vi "FMV - click on control.vi"(8 "error in (no error)":errorcluster, 10 "Reference to Button":refnum<vi>, 11 "VI Reference":refnum<vi>) -> (0 "error out":errorcluster)   [LabVIEW 2020, in "ui-testing.lvlib"]
uses:
  ui-testing.lvlib
  User32.dll
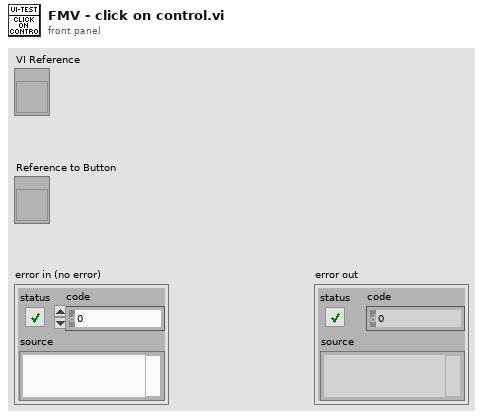
[diagram p1: front panel]
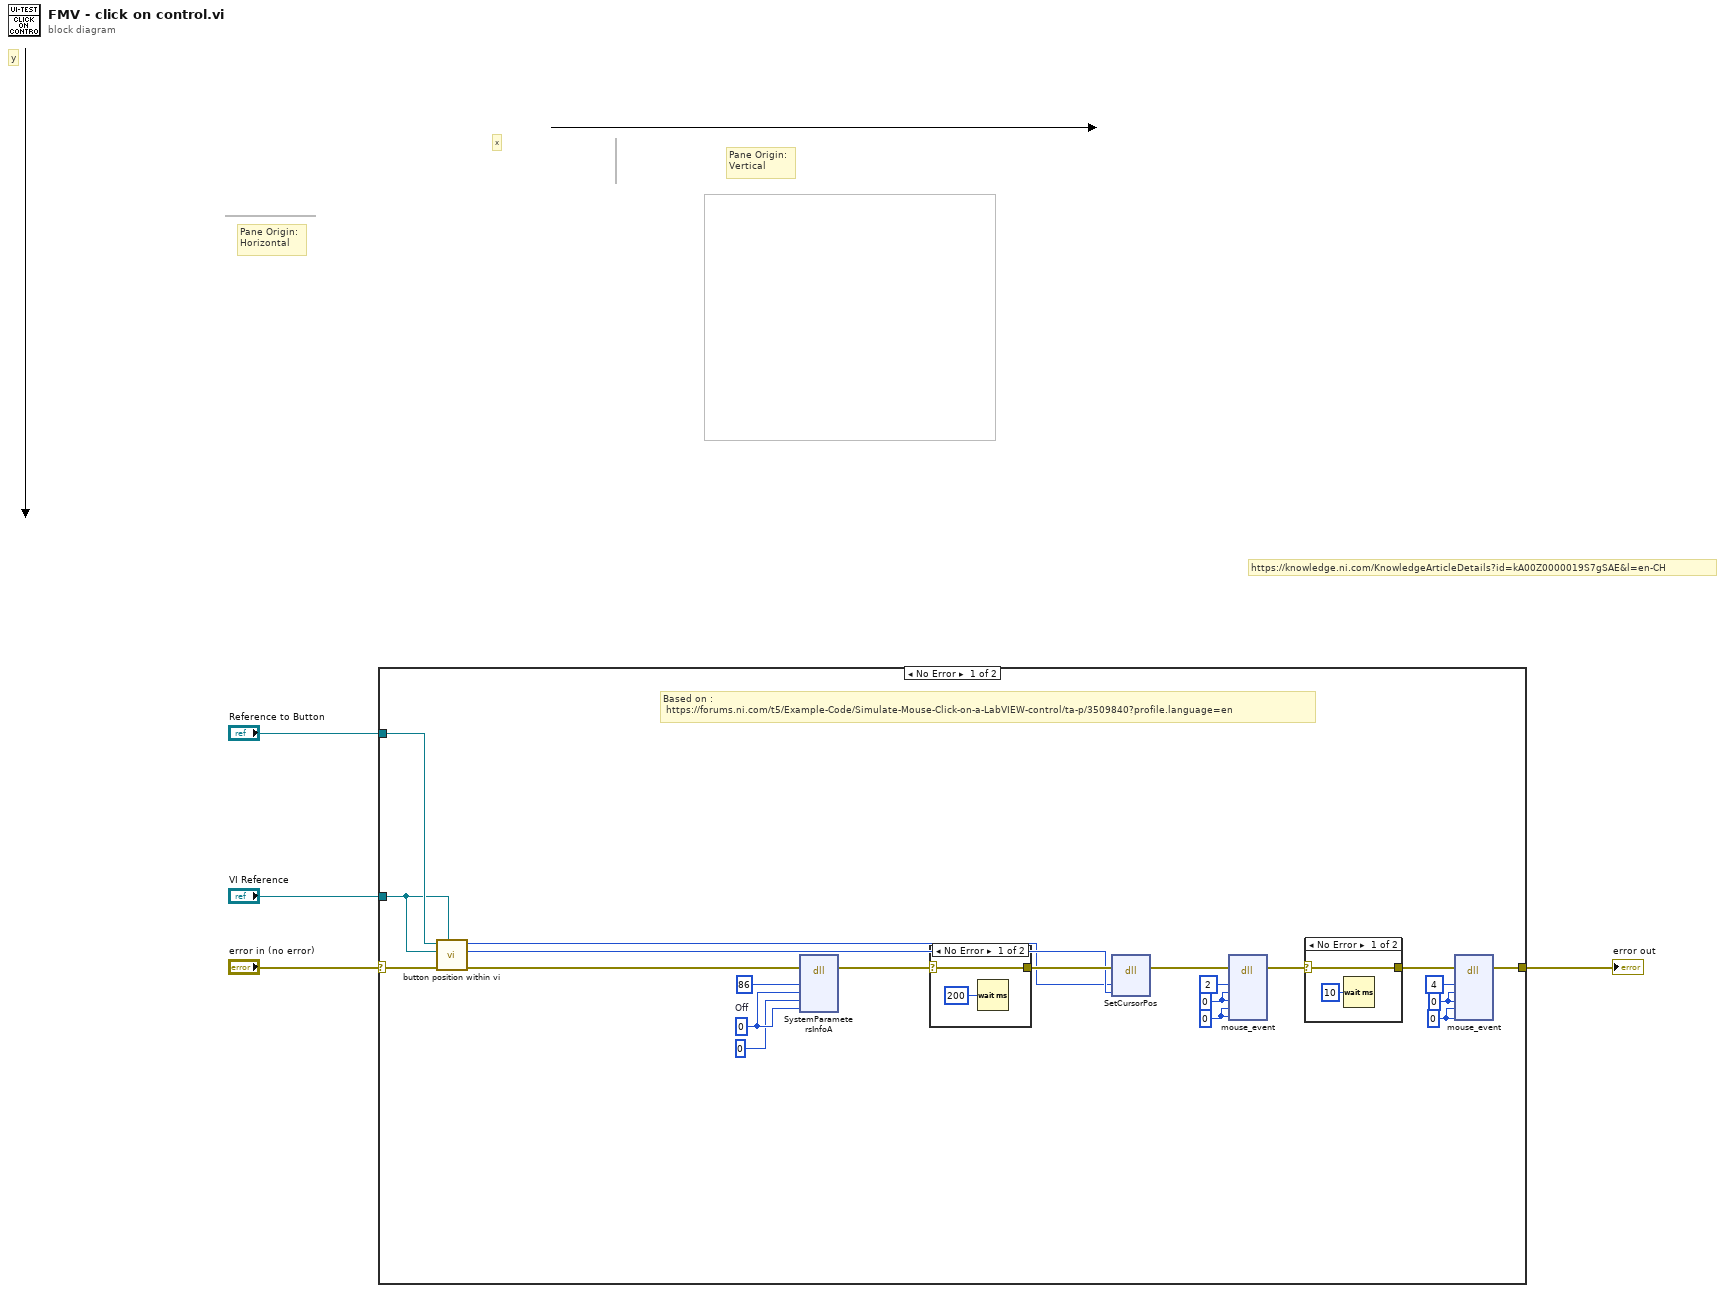
[diagram p0: block diagram]
diagram:
  # "https://knowledge.ni.com/KnowledgeArticleDetails?id=kA00Z0000019S7gSAE&l=en-CH"
  # "Pane Origin:\nVertical"
  # "Pane Origin:\nHorizontal"
  # "y"
  # "x"
  n1 = case shown="No Error" "error in (no error)" {
    selector: "error in (no error)" -> [w8 w32]
    tunnel: [w11 w32] -> w4
    tunnel: "Reference to Button" -> [w6 _]
    tunnel: "VI Reference" -> [w5 _]
    frame No Error {
      w23 = 0 ("dwExtraInfo")
      w24 = u32 0 ("dwExtraInfo")
      w22 = 0 ("dwExtraInfo")
      w21 = u32 0 ("dwExtraInfo")
      w19 = u32 0  # Off
      # "Based on :\n https://forums.ni.com/t5/Example-Code/Simulate-Mouse-Click-on-a-LabVIEW-control/ta-p/3509840?profile.language=en"
      n2 = call "button position within vi.vi"("VI with focus"=w5, "error in (no error)"=w8, "VI Reference"=w5, "Boolean in"=w6) -> ("error out"=w7:errorcluster, "Vertical"=w10:i16, "Horizontal"=w9:i16)  [unwired: 3 in, 2 out]
      n3 = dll-call lib="User32.dll" fn="SystemParametersInfoA" label="Terminate power-off mode"(error in=w7, "uiAction"=u32 86 ("SPI_GETPOWEROFFACTIVE"), "uiParam"=w19, "pvParam"=0, "fWinIni"=w19) -> (error out=w16:errorcluster)  [unwired: 7 in, 1 out]
      n4 = case shown="No Error" w16 {
        selector: w16 -> [w29 w31]
        tunnel: [w29 w31] -> w15
        frame No Error {
          n5 = Wait (ms)(milliseconds to wait=u32 200) -> ()  [unwired: 1 out]
        }
        frame Error {
        }
      }
      n6 = dll-call lib="User32.dll" fn="SetCursorPos" label="Move mouse"(error in=w15, "dx"=w9, "dy"=w10) -> (error out=w14:errorcluster)  [unwired: 5 in, 1 out]
      n7 = dll-call lib="User32.dll" fn="mouse_event" label="Click"(error in=w14, "dwFlags"=2, "dx"=w22, "dy"=w22, "dwData"=w21, "dwExtraInfo"=w21) -> (error out=w13:errorcluster)  [unwired: 8 in, 1 out]
      n8 = case shown="No Error" w13 {
        selector: w13 -> [w26 w28]
        tunnel: [w26 w28] -> w12
        frame No Error {
          n9 = Wait (ms)(milliseconds to wait=u32 10) -> ()  [unwired: 1 out]
        }
        frame Error {
        }
      }
      n10 = dll-call lib="User32.dll" fn="mouse_event" label="Release"(error in=w12, "dwFlags"=4, "dx"=w23, "dy"=w23, "dwData"=w24, "dwExtraInfo"=w24) -> (error out=w11:errorcluster)  [unwired: 8 in, 1 out]
    }
    frame Error {
    }
  }
  "error out" <- w4
